vi "CVT Double Read.vi"(3 "error in (no error)":errorcluster, 5 "Tag Name":string) -> (0 "error out":errorcluster, 1 "Value":dbl)   [LabVIEW 2020, in "Current Value Table(Rebuild).lvlib"]
uses:
  Current Value Table(Rebuild).lvlib
  DataTypes/Double_Read.vi
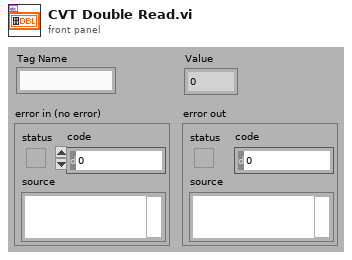
[diagram p1: front panel]
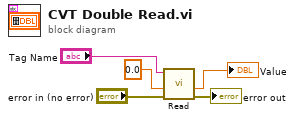
[diagram p0: block diagram]
diagram:
  n1 = call-poly "Read.vi"("error in (no error)"="error in (no error)", "Default"=0.0, "Tag Name"="Tag Name") -> ("error out"=→"error out":errorcluster, "Value"=→"Value":dbl)  [unwired: 7 in]
